vi "Expt_5_Receiver_1.vi"() -> ()   [LabVIEW 2022 SP3]
uses:
  <instrlib>/niUSRP/niUSRP Fetch Rx Data (CDB).vi
  <vilib>/Analysis/NI_AALPro.lvlib
panel:
  out "Demodulated":dbl[](graph)
  out "XY Graph":cluster{i32[], i32[]}(graph)
  out "Array 4":i32[](array[numeric])
  out "Array 3":i32[](array[numeric])
  in  "stop":bool
  in  "active antenna 2":string
  in  "gain 2":dbl format="%#_6f"
  in  "carrier frequency 2":dbl=100000.0 format="%#_6p"
  in  "IQ rate 2":dbl=100000.0 format="%#_6p"
  in  "device names 2":refnum<k15>
  out "Array 2":dbl[](array[numeric])
  in  "active antenna":string
  in  "gain":dbl format="%#_6f"
  in  "carrier frequency":dbl=100000.0 format="%#_6p"
  in  "IQ rate":dbl=100000.0 format="%#_6p"
  in  "device names":refnum<k15>
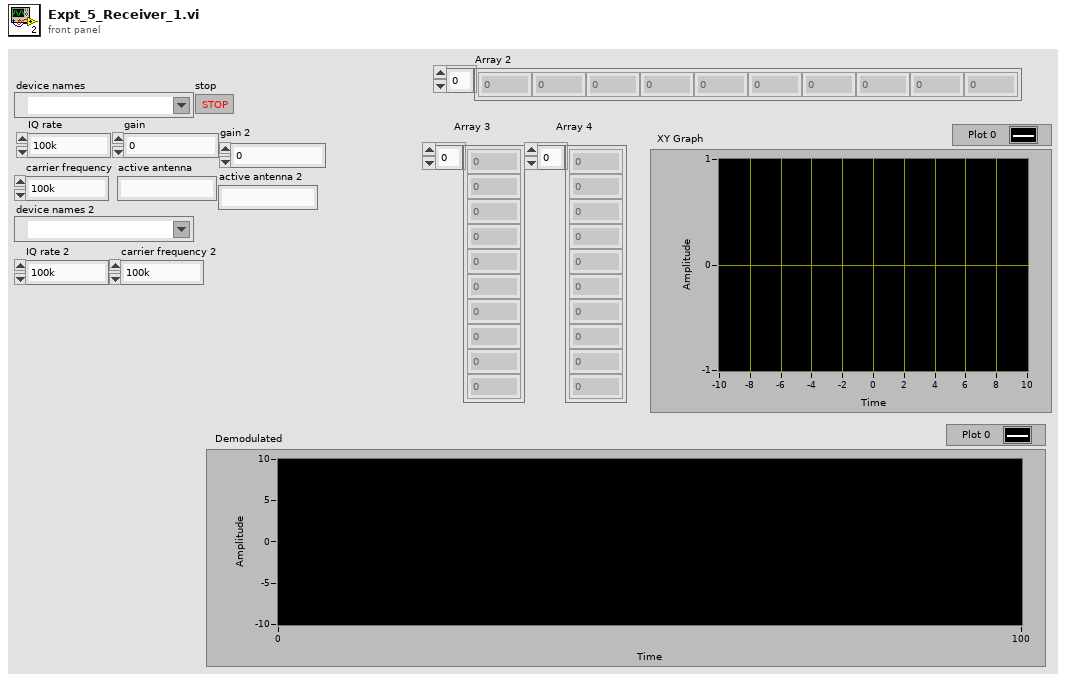
[diagram p1: front panel]
types:
  T1 = enum16{"sine", "cosine", "triangle", "square", "sawtooth", "increasing ramp", "decreasing ramp"}
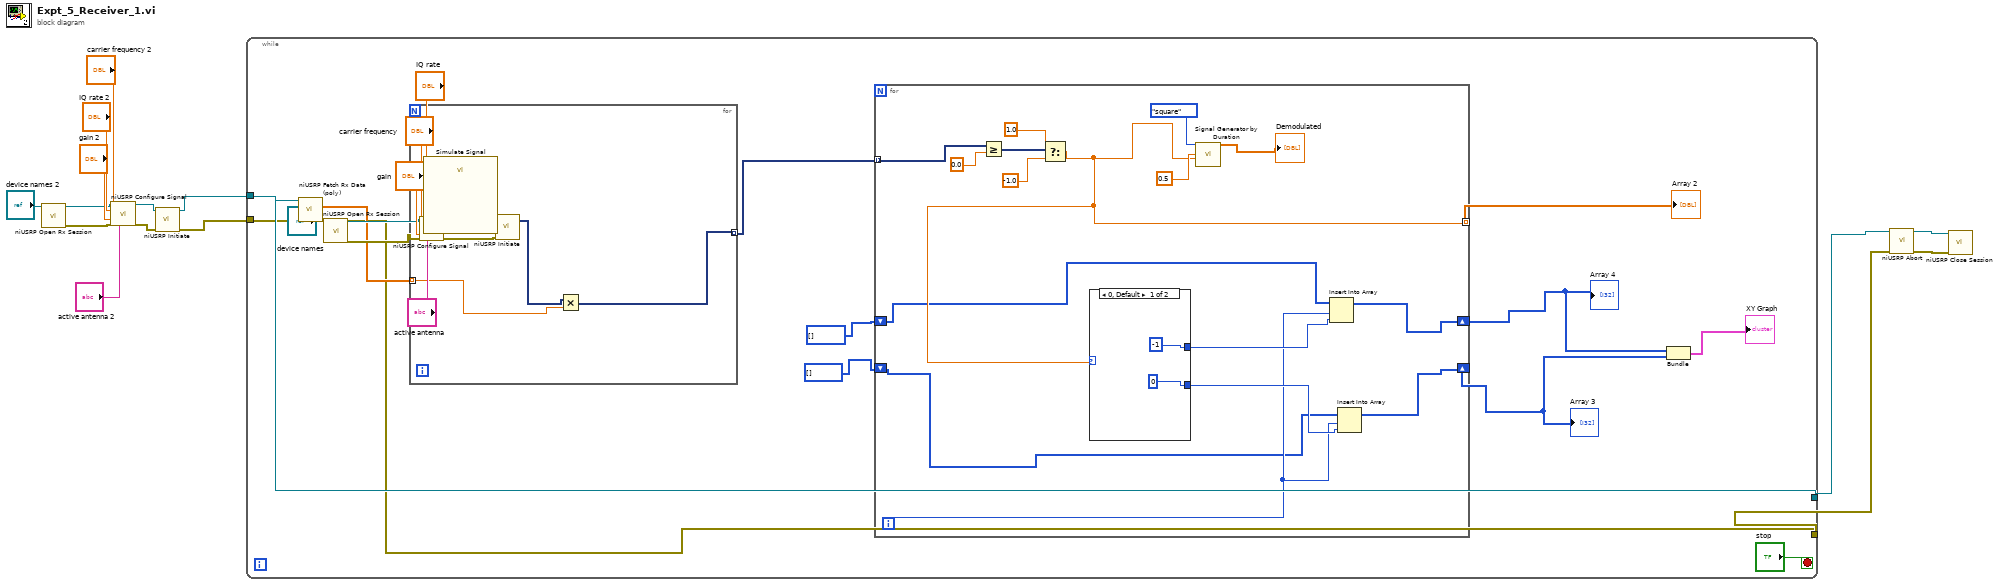
[diagram p0: block diagram]
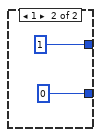
[diagram p2: hidden frame]
diagram:
  n1 = call <instrlib>:"niUSRP Open Rx Session.vi"("device names"="device names 2") -> ("session handle out"=w6:refnum<k15>, "error out"=w5:errorcluster)  [unwired: 13 in]
  n2 = call <instrlib>:"niUSRP Configure Signal.vi"("session handle"=w6, "IQ rate"="IQ rate 2", "carrier frequency"="carrier frequency 2", "gain"="gain 2", "error in (no error)"=w5, "active antenna"="active antenna 2") -> ("session handle out"=w7:refnum<k15>, "error out"=w4:errorcluster)  [unwired: 5 in, 3 out]
  n3 = call <instrlib>:"niUSRP Initiate.vi"("session handle"=w7, "error in (no error)"=w4) -> ("session handle out"=w2:refnum<k15>, "error out"=w1:errorcluster)  [unwired: 12 in]
  n4 = while {
    tunnel: [w34] -> w13
    tunnel: [w33] -> w12
    tunnel: w2 -> [w32]
    tunnel: w1 -> [w31]
    stop <- "stop" stop-if-true
    n5 = call-poly <instrlib>:"niUSRP Fetch Rx Data (poly).vi"("session handle"=w32, "error in (no error)"=w31) -> ("session handle out"=w34:refnum<k15>, "data"=w35:cdb[], "error out"=w33:errorcluster)  [unwired: 10 in, 1 out]
    n6 = for {
      tunnel: [w59] -> w37 mode=indexing
      tunnel: w35 -> [w58] mode=indexing
      n7 = call "Simulate Signal"() -> ("Cos"=w60:dynamicdata)  [unwired: 14 in, 1 out]
      n8 = Multiply(x=w60, y=w58) -> (x*y=w59:dynamicdata)
    }
    n9 = for {
      tunnel: w37 -> [w52] mode=indexing
      tunnel: [w44] -> w36 mode=indexing
      shift-right: [w40] -> w26
      shift-left: i32[] [] -> [w42]
      shift-right: [w39] -> w25
      shift-left: i32[] [] -> [w41]
      i -> [w43]
      n10 = Greater Or Equal?(x=w52, y=0.0) -> (x >= y?=w47:dynamicdata)
      n11 = Select(t=1.0, s=w47, f=-1.0) -> (s? t:f=w44:dbl)
      n12 = case shown="0, Default" w44 {
        tunnel: [-1 1] -> w46
        tunnel: [0 0] -> w45
        frame 0, Default {
        }
        frame 1 {
        }
      }
      n13 = call <vilib>:"Signal Generator by Duration.vi"("signal type"=T1."square", "frequency"=0.5, "amplitude"=w44) -> ("signal"=→"Demodulated":dbl[])  [unwired: 9 in, 3 out]
      n14 = Insert Into Array(array=w42, index=w43, new element=w46) -> (w40:i32[])
      n15 = Insert Into Array(array=w41, index=w43, new element=w45) -> (w39:i32[])
    }
    "Array 2" <- w36
    "Array 3" <- w25
    "Array 4" <- w26
    n16 = Bundle(w26, w25) -> (→"XY Graph":cluster{i32[], i32[]})  [unwired: 1 in]
  }
  n17 = call <instrlib>:"niUSRP Open Rx Session.vi"("device names"="device names") -> ("session handle out"=w19:refnum<k15>, "error out"=w18:errorcluster)  [unwired: 13 in]
  n18 = call <instrlib>:"niUSRP Configure Signal.vi"("session handle"=w19, "IQ rate"="IQ rate", "carrier frequency"="carrier frequency", "gain"="gain", "error in (no error)"=w18, "active antenna"="active antenna") -> ("session handle out"=w17:refnum<k15>, "error out"=w16:errorcluster)  [unwired: 5 in, 3 out]
  n19 = call <instrlib>:"niUSRP Initiate.vi"("session handle"=w17, "error in (no error)"=w16) -> ()  [unwired: 12 in, 2 out]
  n20 = call <instrlib>:"niUSRP Abort.vi"("session handle"=w13, "error in (no error)"=w12) -> ("session handle out"=w15:refnum<k15>, "error out"=w14:errorcluster)  [unwired: 12 in]
  n21 = call <instrlib>:"niUSRP Close Session.vi"("session handle"=w15, "error in (no error)"=w14) -> ()  [unwired: 13 in, 1 out]
